vi "Save Front Panel Window Position.vi"(8 "error in (no error)":errorcluster, 11 "Actor in":refnum<class "Actor.lvclass">) -> (0 "error out":errorcluster)   [LabVIEW 2021, in "Actor.lvclass"]
uses:
  Actor.lvclass
  Actor.lvclass/Actor.ctl
  <userlib>/_OpenG.lib/variantconfig/variantconfig.llb/openg_variant_configuration_file.lvlib
  <vilib>/Utility/config.llb/NI_LVConfig.lvlib
  <vilib>/Utility/miscctls.llb/LVRectTypeDef.ctl
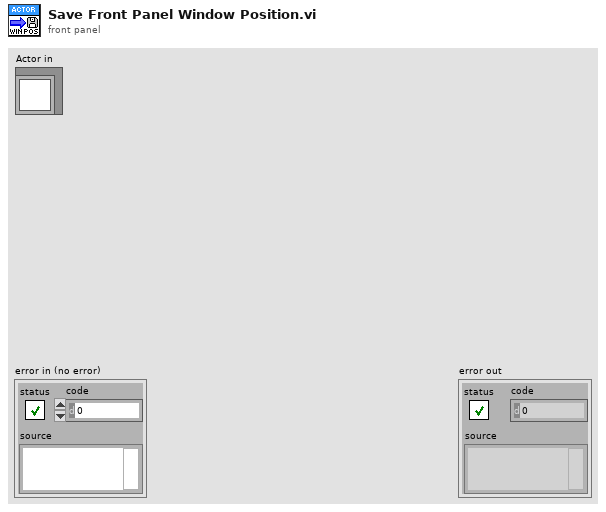
[diagram p1: front panel]
types:
  T1 = typedef "LVRectTypeDef.ctl" = cluster{"Left":i16, "Top":i16, "Right":i16, "Bottom":i16}
  T2 = typedef "NI_LVConfig.lvlib/Config Data RefNum.ctl" = refnum<k1>
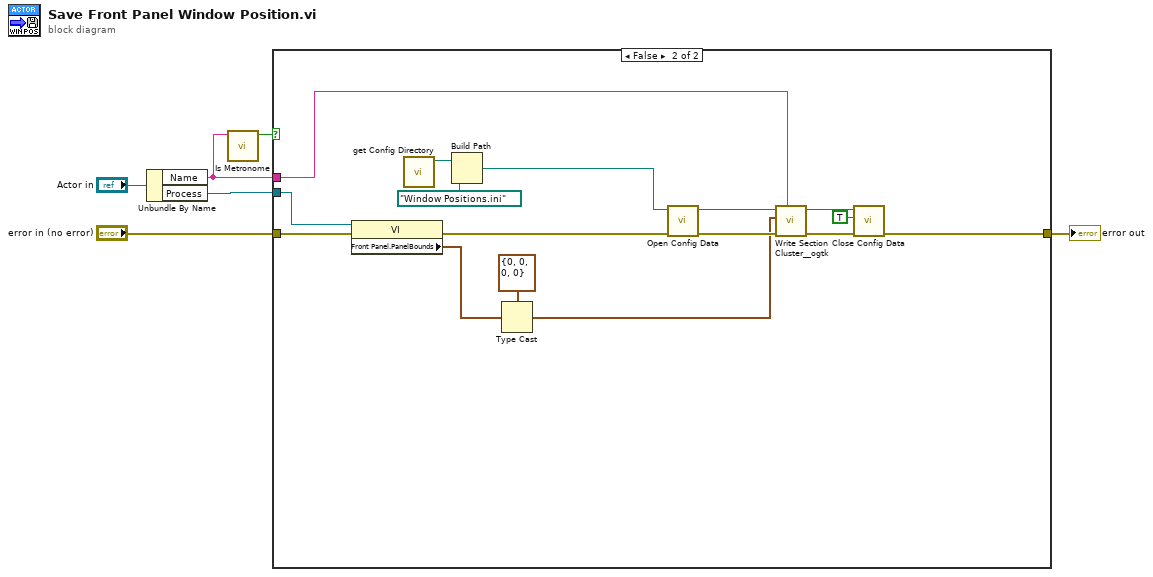
[diagram p0: block diagram]
diagram:
  n1 = Unbundle By Name("Actor in") -> ("Name"=w1:string, "Process"=w6:refnum<vi>)
  n2 = call "Is Metronome.vi"("Actor Name"=w1) -> ("Is Metronome"=w2:bool)  [unwired: 10 in]
  n3 = case shown="False" w2 {
    tunnel: w6 -> [_ w19]
    tunnel: "error in (no error)" -> [w7 w18]
    tunnel: [w7 w14] -> w3
    tunnel: w1 -> [_ w8]
    frame True {
      # "Do not bother saving positions of Metronomes"
    }
    frame False {
      n4 = property class="VI"(reference=w19, error in=w18) -> (error out=w9:errorcluster, "Front Panel.PanelBounds"=w22:T1)  [unwired: 1 out]
      n5 = call "get Config Directory.vi"() -> ("Config Dir"=w10:path)  [unwired: 11 in]
      n6 = Build Path(base path=w10, name or relative path=path "Window Positions.ini" ("configuration file path")) -> (appended path=w12:path)
      n7 = Type Cast(type=T1 {"Left"=0, "Top"=0, "Right"=0, "Bottom"=0} ("Front Panel Window:Panel Bounds"), x=w22) -> (*(type *) &x=w11:T1)
      n8 = call <vilib>:"Open Config Data.vi"("error in (no error)"=w9, "configuration file path"=w12) -> ("error out"=w20:errorcluster, "refnum"=w21:T2)  [unwired: 7 in, 1 out]
      n9 = call <userlib>:"Write Section Cluster__ogtk.vi"("section (optional)"=w8, "error in (no error)"=w20, "Section Formatted Cluster"=w11, "refnum"=w21) -> ("error out"=w16:errorcluster, "dup refnum"=w15:T2)  [unwired: 6 in]
      n10 = call <vilib>:"Close Config Data.vi"("error in (no error)"=w16, "write file if changed (T)"=TRUE, "refnum"=w15) -> ("error out"=w14:errorcluster)  [unwired: 7 in, 1 out]
    }
  }
  "error out" <- w3
